vi "Parse Error XML.vi"(9 "Code Tag Value":string, 10 "Error XML":string, 11 "AWS Core":refnum<class "Queue.lvclass">) -> (1 "Error Description":string, 2 "Error Code":i32, 3 "Warning":bool)   [LabVIEW 2015, in "NI_AWS_SQS.lvlib" / "Queue.lvclass"]
uses:
  Queue.lvclass
  Core/HTTP Request/HTTP Request.lvclass
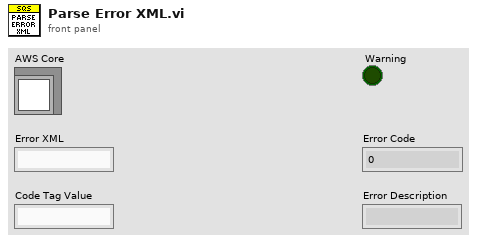
[diagram p1: front panel]
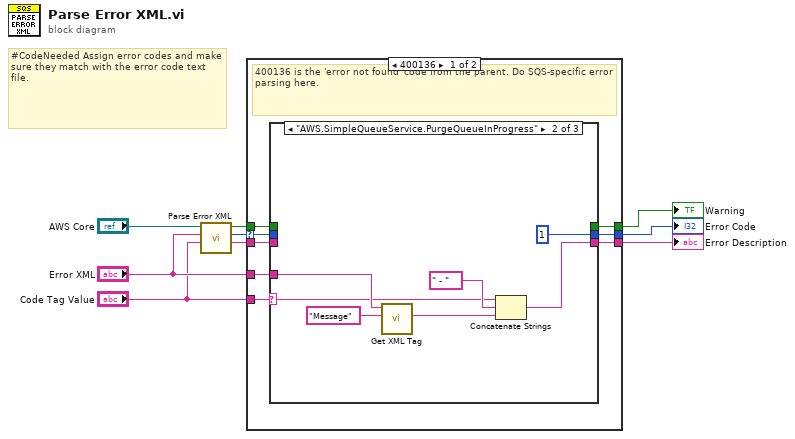
[diagram p0: block diagram]
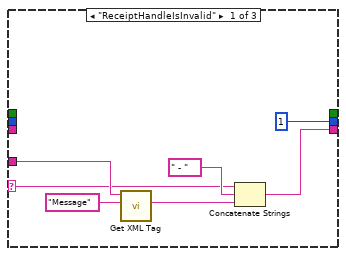
[diagram p2: hidden frame]
diagram:
  # "#CodeNeeded Assign error codes and make sure they match with the error code text file."
  n1 = call-parent "Parse Error XML.vi"("Code Tag Value"="Code Tag Value", "Error XML"="Error XML", "AWS Core"="AWS Core") -> ("Error Description"=w6:string, "Error Code"=w8:i32, "Warning"=w7:bool)  [unwired: 6 in]
  n2 = case shown="400136" w8 {
    selector: w8 -> [w14 w35]
    tunnel: w7 -> [w15 w37]
    tunnel: w6 -> [w13 w36]
    tunnel: [w12 w37] -> w5
    tunnel: [w10 w36] -> w4
    tunnel: [w11 w35] -> w3
    tunnel: "Error XML" -> [w17 _]
    tunnel: "Code Tag Value" -> [w16 _]
    frame 400136 {
      # "400136 is the 'error not found' code from the parent. Do SQS-specific error parsing here."
      n3 = case shown="\"AWS.SimpleQueueService.PurgeQueueInProgress\"" w16 {
        selector: w16 -> [w18 w25 _]
        tunnel: w17 -> [w19 w26 _]
        tunnel: w15 -> [_ _ w34]
        tunnel: w14 -> [_ _ w33]
        tunnel: w13 -> [_ _ w32]
        tunnel: [_ _ w34] -> w12
        tunnel: [1 1 w33] -> w11
        tunnel: [w20 w27 w32] -> w10
        frame "ReceiptHandleIsInvalid" {
          n4 = call "Get XML Tag.vi"("Tag name"="Message", "XML String in"=w19) -> ("Tag value"=w22:string)  [unwired: 5 in, 4 out]
          n5 = Concatenate Strings(w18, " - " ("string"), w22) -> (w20:string)
        }
        frame "AWS.SimpleQueueService.PurgeQueueInProgress" {
          n6 = call "Get XML Tag.vi"("Tag name"="Message", "XML String in"=w26) -> ("Tag value"=w29:string)  [unwired: 5 in, 4 out]
          n7 = Concatenate Strings(w25, " - " ("string"), w29) -> (w27:string)
        }
        frame Default {
          # "Unknown error code, use default error from parent"
        }
      }
    }
    frame Default {
      # "Parent method already assigned an error code"
    }
  }
  "Error Description" <- w4
  "Warning" <- w5
  "Error Code" <- w3
